vi "Auto ROI Setting UI.vi"() -> ()   [LabVIEW 2015]
uses:
  Controls/AutoROIMode.ctl
  Controls/AutoROIPage.ctl
  Controls/AutoROIUI.ctl
  <vilib>/Utility/miscctls.llb/LVPointTypeDef.ctl
panel:
  in  "ROI List":i32[](listbox)
  out "ModeTab":T1
  in  "Numbers":i32=1 min=1 step=1
  in  "X Pitch":i32
  in  "X Numbers":i32
  in  "Y Pitch":i32
  in  "Y Numbers":i32
  in  "Step":u16(ring) items=["1 pixel"=1, "10 pixel"=10, "100 pixel"=100]
  in  "X+":bool
  in  "X-":bool
  in  "Y-":bool
  in  "Y+":bool
  in  "Add":bool
  in  "Mode":T2
  in  "Cancel":bool
  in  "OK":bool
  out "Vision_Image":T3(plugin-control)
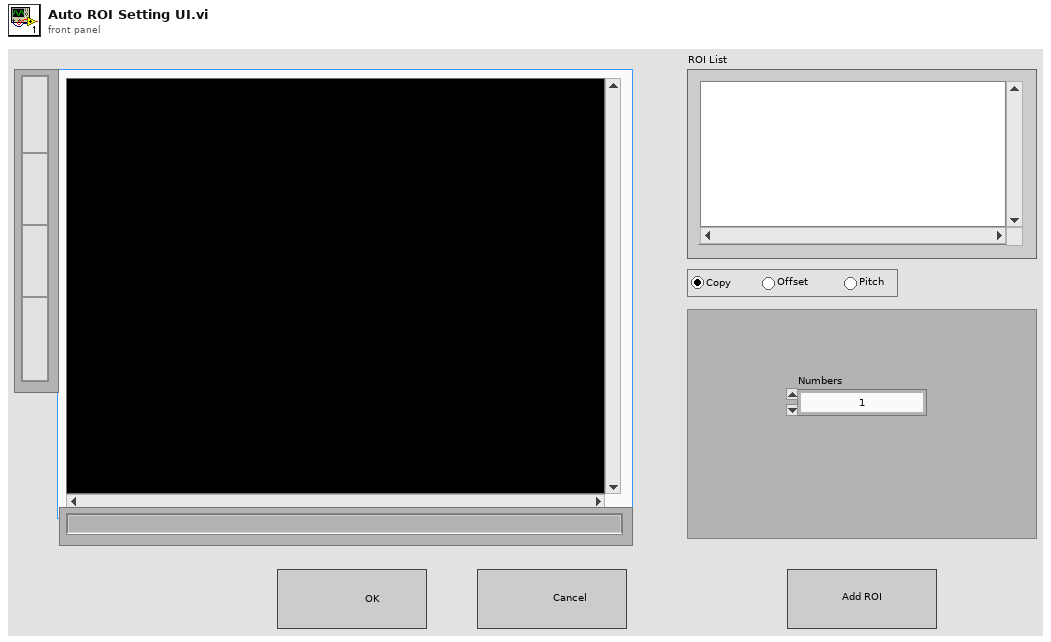
[diagram p1: front panel]
types:
  T1 = typedef "AutoROIPage.ctl" = enum32{"Copy", "Pitch", "Offset"}
  T2 = typedef "AutoROIMode.ctl" = enum32{"Copy", "Pitch", "Offset"}
  T3 = typedef "IMAQ Image.ctl" = refnum<image>
  T4 = typedef "LVPointTypeDef.ctl" = cluster{"Horizontal":i16, "Vertical":i16}
  T5 = typedef "AutoROIUI.ctl" = cluster{"Message":enum16{"Initialize", "UpdateROIList", "UpdateROI", "Add", "Move", "OK", "Cancel", "Exit"}, "Data":variant}
  T6 = enum8{"Enabled", "Disabled", "Disabled and Grayed Out"}
  T7 = enum16{"Initialize", "UpdateROIList", "UpdateROI", "Add", "Move", "OK", "Cancel", "Exit"}
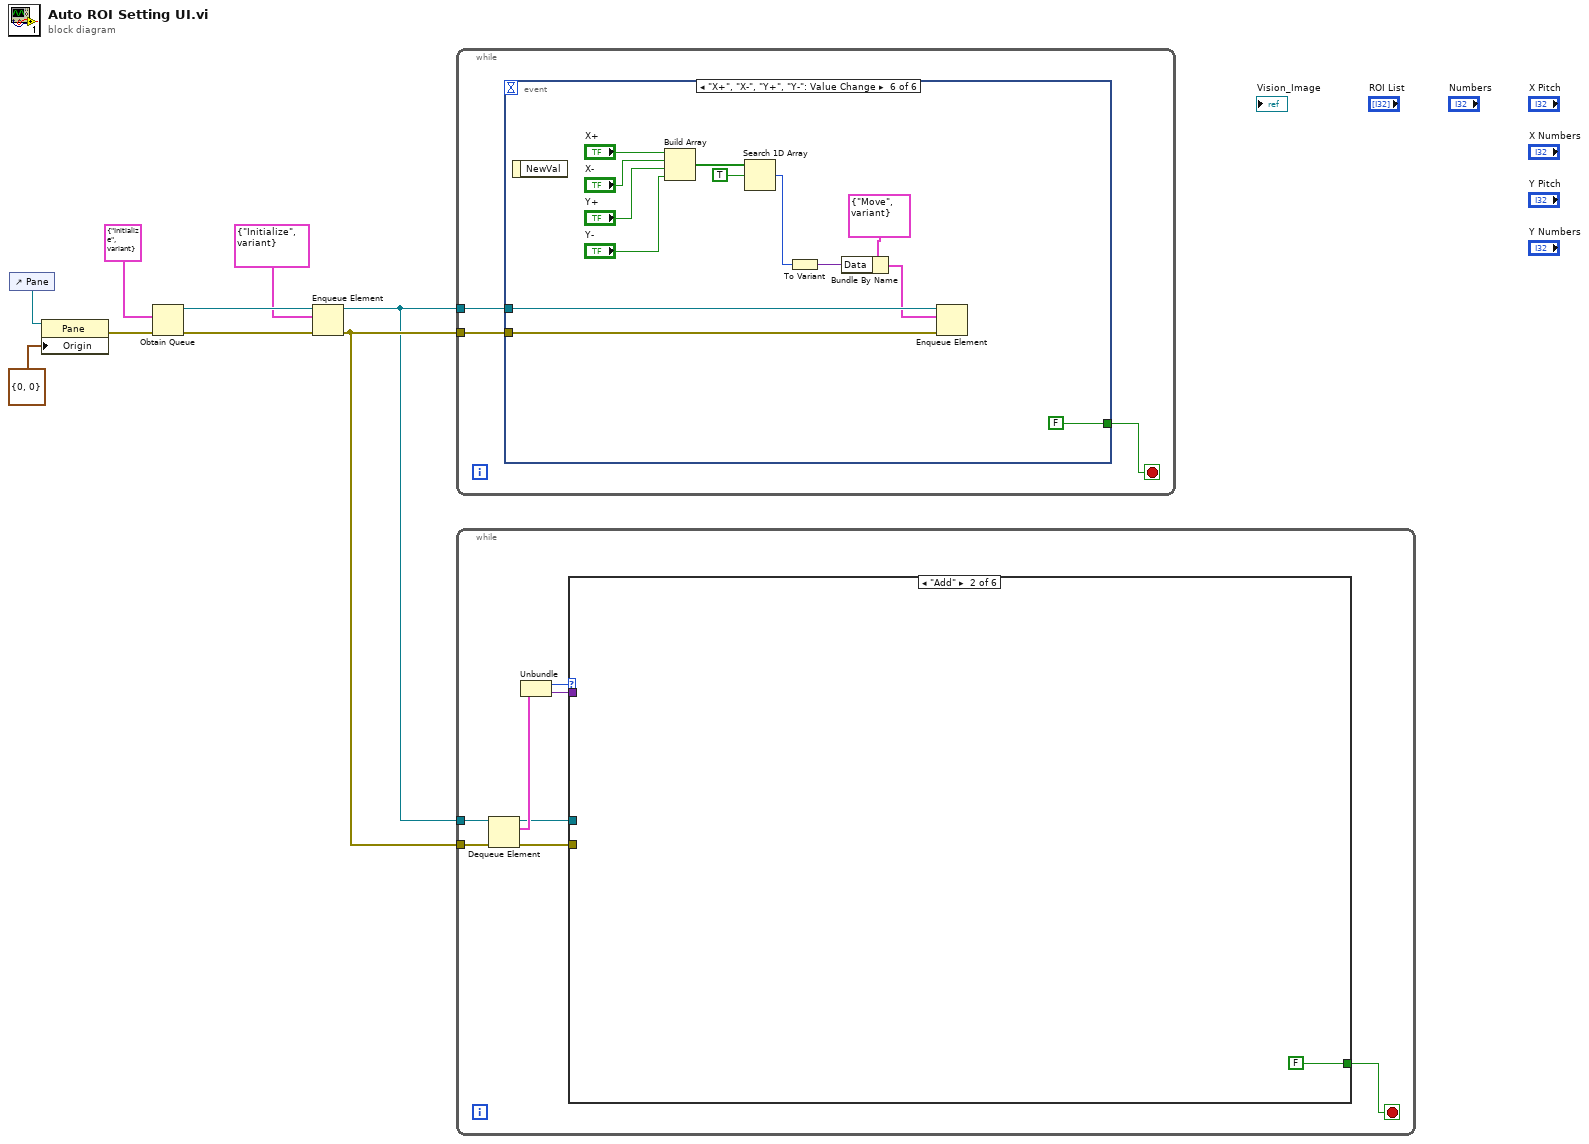
[diagram p0: block diagram]
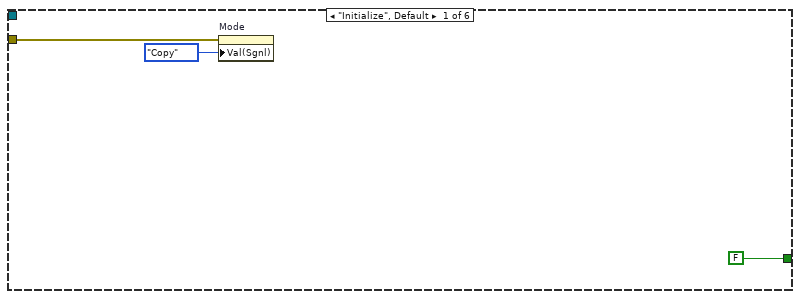
[diagram p2: hidden frame]
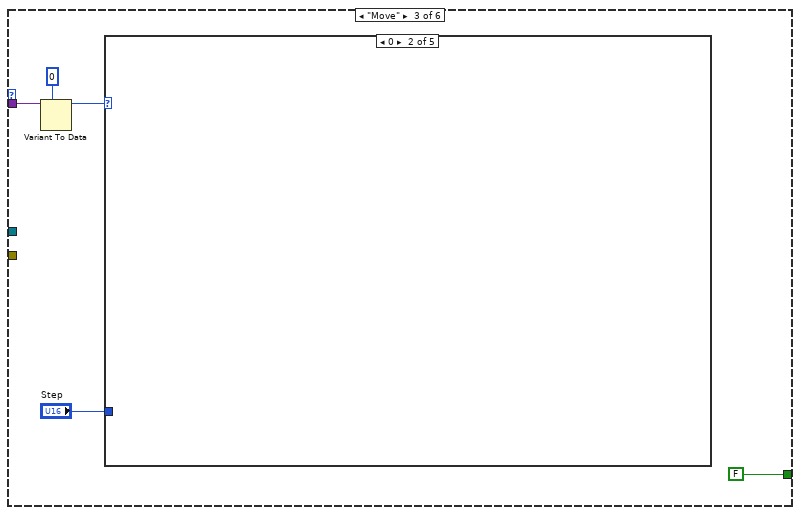
[diagram p3: hidden frame]
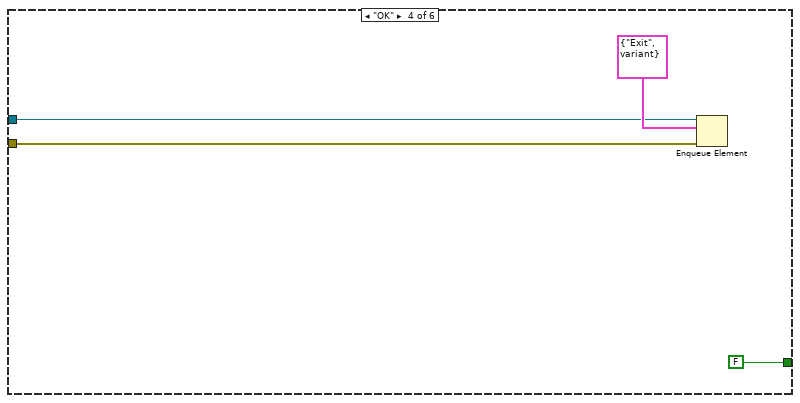
[diagram p8: hidden frame]
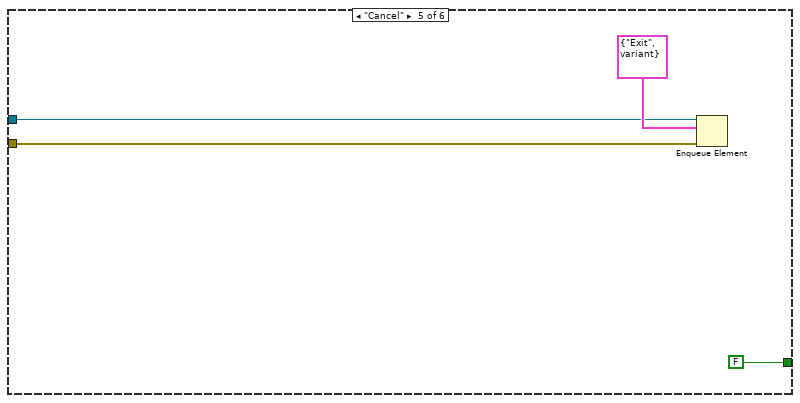
[diagram p9: hidden frame]
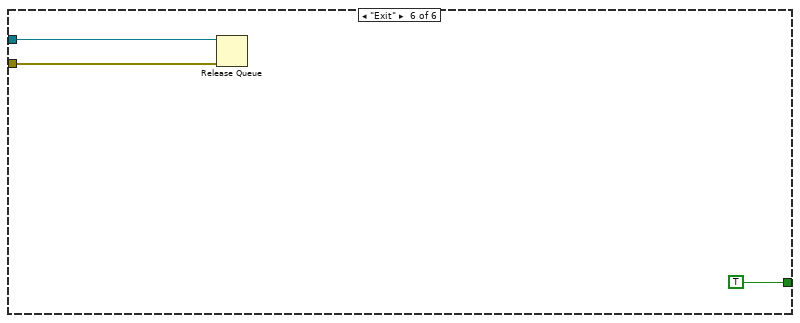
[diagram p10: hidden frame]
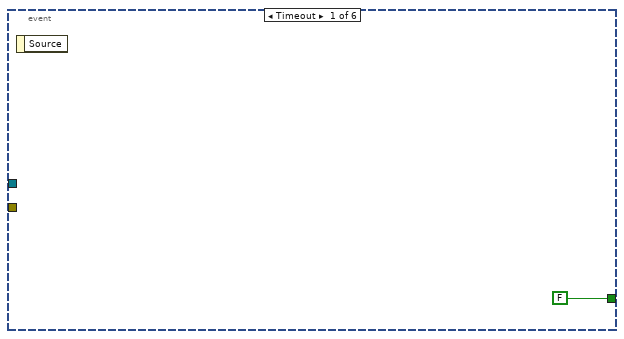
[diagram p11: hidden frame]
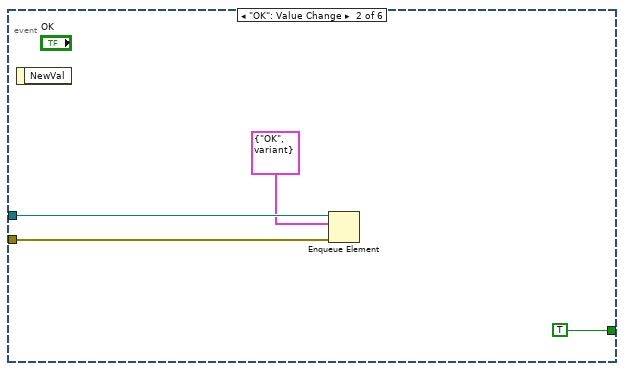
[diagram p12: hidden frame]
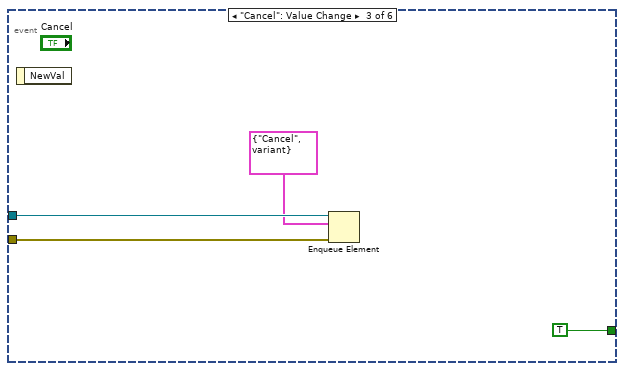
[diagram p13: hidden frame]
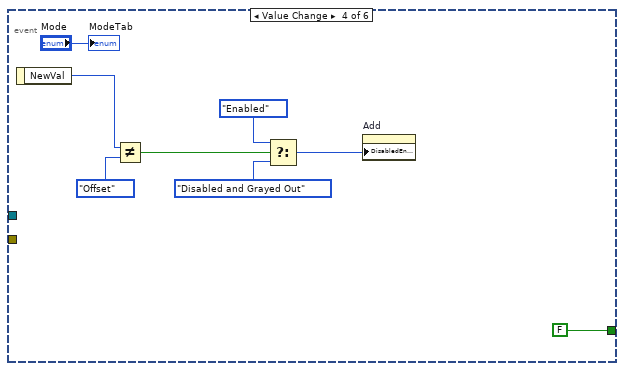
[diagram p14: hidden frame]
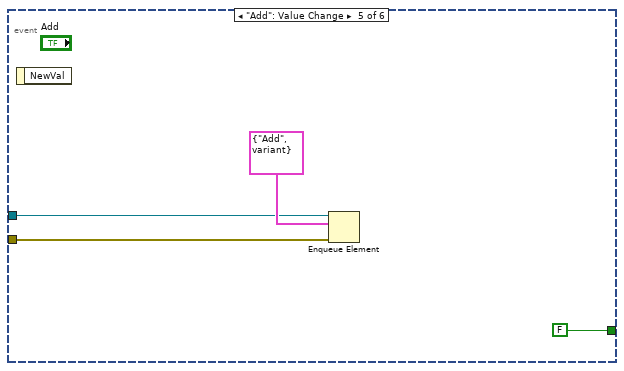
[diagram p15: hidden frame]
diagram:
  n1 = control-ref of="Pane"() -> (w3:refnum<vi>)
  n2 = property class="Pane"(reference=w3, "Origin"=T4 {"Horizontal"=0, "Vertical"=0}) -> (error out=w2:errorcluster)  [unwired: 1 in, 1 out]
  n3 = Obtain Queue(element data type=T5 {"Message"=enum."Initialize", "Data"=variant} ("AutoROIUI"), error in (no error)=w2) -> (queue out=w9:refnum<queue>, error out=w8:errorcluster)  [unwired: 3 in, 1 out]
  n4 = Enqueue Element(queue=w9, element=T5 {"Message"=enum."Initialize", "Data"=variant}, error in (no error)=w8) -> (queue out=w4:refnum<queue>, error out=w5:errorcluster)  [unwired: 1 in, 1 out]
  n5 = while {
    tunnel: w4 -> [w11]
    tunnel: w5 -> [w10]
    stop <- w12 stop-if-true
    n6 = event shown="[5] \"X+\", \"X-\", \"Y+\", \"Y-\": Value Change" {
      selector: _ -> [_ _ _ _ _ _]
      dyn-events: _ -> [_ _ _ _ _ _]
      timeout: _ -> [_ _ _ _ _ _]
      tunnel: [FALSE TRUE TRUE FALSE FALSE FALSE] -> w12
      tunnel: w11 -> [_ w16 w20 _ w31 w40]
      tunnel: w10 -> [_ w15 w19 _ w30 w39]
      event Timeout {
        n7 = event-data() -> ()  [unwired: 1 in, 1 out]
      }
      event "OK": Value Change {
        n8 = event-data() -> ()  [unwired: 1 in, 1 out]
        n9 = Enqueue Element(queue=w16, element=T5 {"Message"=enum."OK", "Data"=variant}, error in (no error)=w15) -> ()  [unwired: 1 in, 3 out]
      }
      event "Cancel": Value Change {
        n10 = event-data() -> ()  [unwired: 1 in, 1 out]
        n11 = Enqueue Element(queue=w20, element=T5 {"Message"=enum."Cancel", "Data"=variant}, error in (no error)=w19) -> ()  [unwired: 1 in, 3 out]
      }
      event Value Change {
        n12 = event-data() -> ("NewVal"=w25:T2)  [unwired: 1 in]
        n13 = Not Equal?(x=w25, y=AutoROIMode."Offset") -> (x != y?=w26:bool)
        n14 = Select(t=T6."Enabled" ("Disabled"), s=w26, f=T6."Disabled and Grayed Out" ("Disabled")) -> (s? t:f=w22:T6)
        n15 = property on="Add" class="Bool"("DisabledEnum"=w22) -> ()  [unwired: 2 in, 2 out]
        "ModeTab" <- "Mode"
      }
      event "Add": Value Change {
        n16 = event-data() -> ()  [unwired: 1 in, 1 out]
        n17 = Enqueue Element(queue=w31, element=T5 {"Message"=enum."Add", "Data"=variant}, error in (no error)=w30) -> ()  [unwired: 1 in, 3 out]
      }
      event "X+", "X-", "Y+", "Y-": Value Change {
        n18 = event-data() -> ()  [unwired: 1 in, 1 out]
        n19 = Build Array("X+", "X-", "Y+", "Y-") -> (w42:bool[])
        n20 = Search 1D Array(1D array=w42, element=TRUE) -> (index of element=w36:i32)  [unwired: 1 in]
        n21 = To Variant(anything=w36) -> (Variant=w35:variant)
        n22 = Bundle By Name(cluster=T5 {"Message"=enum."Move", "Data"=variant} ("element"), "Data"=w35) -> (w37:T5)
        n23 = Enqueue Element(queue=w40, element=w37, error in (no error)=w39) -> ()  [unwired: 1 in, 3 out]
      }
    }
  }
  n24 = while {
    tunnel: w5 -> [w54]
    tunnel: w4 -> [w53]
    stop <- w50 stop-if-true
    n25 = Dequeue Element(queue=w53, error in (no error)=w54) -> (queue out=w49:refnum<queue>, element=w52:T5, error out=w48:errorcluster)  [unwired: 1 in, 1 out]
    n26 = Unbundle(w52) -> ("Message"=w51:T7, "Data"=w47:variant)
    n27 = case shown="\"Add\"" w51 {
      tunnel: [FALSE FALSE FALSE FALSE FALSE TRUE] -> w50
      tunnel: w49 -> [_ _ _ w65 w69 w73]
      tunnel: w48 -> [w56 _ _ w64 w68 w72]
      tunnel: w47 -> [_ _ w62 _ _ _]
      frame "Initialize", Default {
        n28 = property on="Mode" class="RadioBtnsControl (strict)"(error in=w56, "Val(Sgnl)"=AutoROIMode."Copy" ("Mode")) -> ()  [unwired: 1 in, 2 out]
      }
      frame "Add" {
      }
      frame "Move" {
        n29 = Variant To Data(type=0 ("index of element"), Variant=w62) -> (data=w59:i32)  [unwired: 1 in, 1 out]
        n30 = case shown="0" w59 {
          tunnel: "Step" -> [_ _ _ _ _]
          frame Default {
          }
          frame 0 {
          }
          frame 1 {
          }
          frame 2 {
          }
          frame 3 {
          }
        }
      }
      frame "OK" {
        n31 = Enqueue Element(queue=w65, element=T5 {"Message"=enum."Exit", "Data"=variant}, error in (no error)=w64) -> ()  [unwired: 1 in, 3 out]
      }
      frame "Cancel" {
        n32 = Enqueue Element(queue=w69, element=T5 {"Message"=enum."Exit", "Data"=variant}, error in (no error)=w68) -> ()  [unwired: 1 in, 3 out]
      }
      frame "Exit" {
        n33 = Release Queue(queue=w73, error in (no error)=w72) -> ()  [unwired: 1 in, 3 out]
      }
    }
  }
